vi "PFS_Telemetry.vi"(10 "Variant":variant) -> (2 "PFS_Telemetry":T1 {"Raw_Telemetry" format="%04x"; "Register_13"."Spare" format="%03x"})   [LabVIEW 2019, in "Variant Parser.lvlib" / "Variant Parser.lvclass"]
uses:
  Library/Variant Parser.lvclass
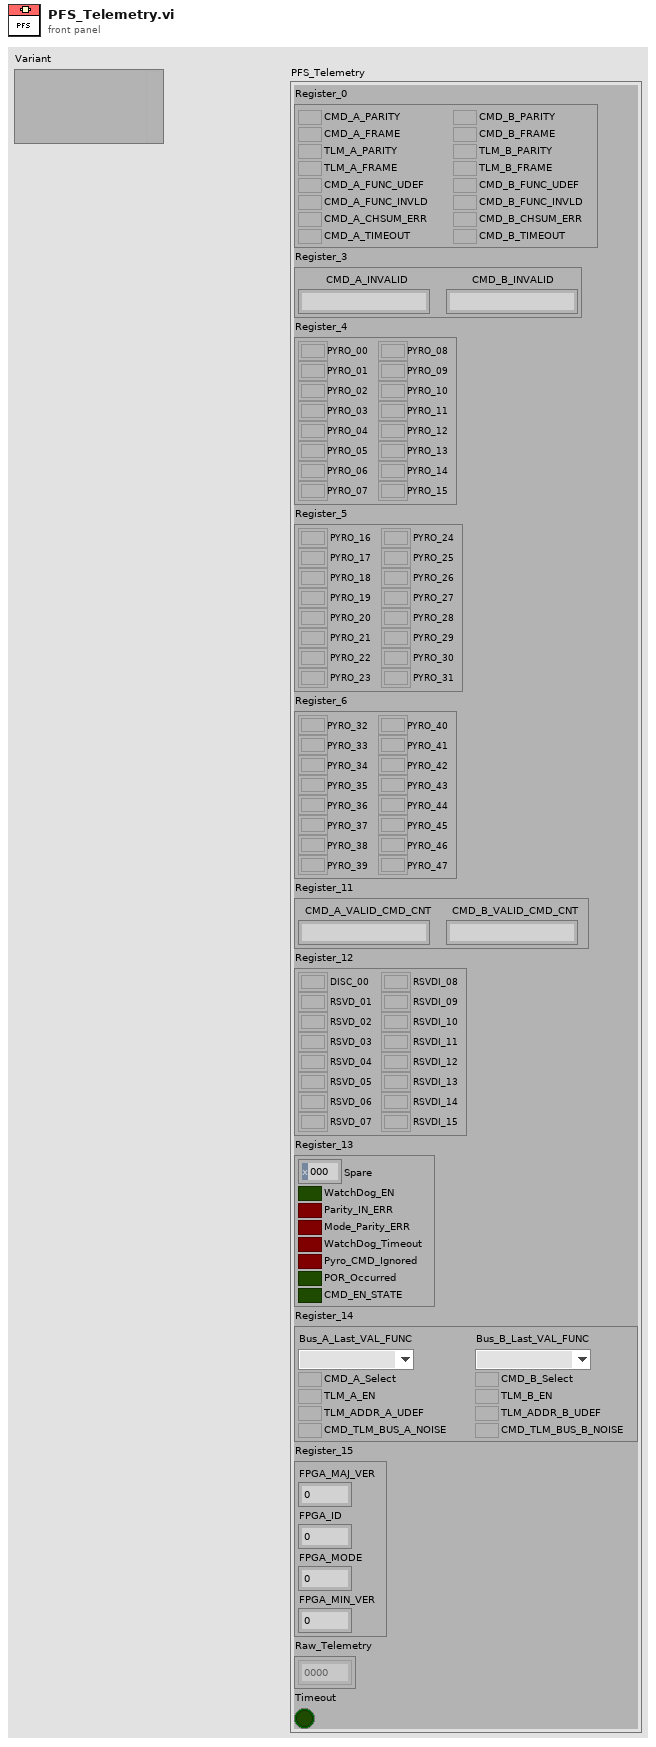
[diagram p1: front panel]
types:
  T1 = cluster{"Register_0":cluster{"CMD_B_PARITY":bool, "CMD_A_PARITY":bool, "CMD_B_FRAME":bool, "CMD_A_FRAME":bool, "TLM_B_PARITY":bool, "TLM_A_PARITY":bool, "TLM_B_FRAME":bool, "TLM_A_FRAME":bool, "CMD_B_FUNC_UDEF":bool, "CMD_A_FUNC_UDEF":bool, "CMD_B_FUNC_INVLD":bool, "CMD_A_FUNC_INVLD":bool, "CMD_B_CHSUM_ERR":bool, "CMD_A_CHSUM_ERR":bool, "CMD_B_TIMEOUT":bool, "CMD_A_TIMEOUT":bool}, "Register_3":cluster{"CMD_B_INVALID":u8, "CMD_A_INVALID":u8}, "Register_4":cluster{"PYRO_00":bool, "PYRO_01":bool, "PYRO_02":bool, "PYRO_03":bool, "PYRO_04":bool, "PYRO_05":bool, "PYRO_06":bool, "PYRO_07":bool, "PYRO_08":bool, "PYRO_09":bool, "PYRO_10":bool, "PYRO_11":bool, "PYRO_12":bool, "PYRO_13":bool, "PYRO_14":bool, "PYRO_15":bool}, "Register_5":cluster{"PYRO_16":bool, "PYRO_17":bool, "PYRO_18":bool, "PYRO_19":bool, "PYRO_20":bool, "PYRO_21":bool, "PYRO_22":bool, "PYRO_23":bool, "PYRO_24":bool, "PYRO_25":bool, "PYRO_26":bool, "PYRO_27":bool, "PYRO_28":bool, "PYRO_29":bool, "PYRO_30":bool, "PYRO_31":bool}, "Register_6":cluster{"PYRO_32":bool, "PYRO_33":bool, "PYRO_34":bool, "PYRO_35":bool, "PYRO_36":bool, "PYRO_37":bool, "PYRO_38":bool, "PYRO_39":bool, "PYRO_40":bool, "PYRO_41":bool, "PYRO_42":bool, "PYRO_43":bool, "PYRO_44":bool, "PYRO_45":bool, "PYRO_46":bool, "PYRO_47":bool}, "Register_11":cluster{"CMD_B_VALID_CMD_CNT":u8, "CMD_A_VALID_CMD_CNT":u8}, "Register_12":cluster{"DISC_00":bool, "RSVD_01":bool, "RSVD_02":bool, "RSVD_03":bool, "RSVD_04":bool, "RSVD_05":bool, "RSVD_06":bool, "RSVD_07":bool, "RSVDI_08":bool, "RSVDI_09":bool, "RSVDI_10":bool, "RSVDI_11":bool, "RSVDI_12":bool, "RSVDI_13":bool, "RSVDI_14":bool, "RSVDI_15":bool}, "Register_13":cluster{"Spare":u16, "WatchDog_EN":bool, "Parity_IN_ERR":bool, "Mode_Parity_ERR":bool, "WatchDog_Timeout":bool, "Pyro_CMD_Ignored":bool, "POR_Occurred":bool, "CMD_EN_STATE":bool}, "Register_14":cluster{"CMD_B_Select":bool, "CMD_A_Select":bool, "TLM_B_EN":bool, "TLM_A_EN":bool, "TLM_ADDR_B_UDEF":bool, "TLM_ADDR_A_UDEF":bool, "CMD_TLM_BUS_B_NOISE":bool, "CMD_TLM_BUS_A_NOISE":bool, "Bus_B_Last_VAL_FUNC":enum16{"No_Command", "IO_Command", "Pyro_Command", "Housekeeping", "Bad_Function"}, "Bus_A_Last_VAL_FUNC":enum16{"No_Command", "IO_Command", "Pyro_Command", "Housekeeping", "Bad_Function"}}, "Register_15":cluster{"FPGA_MAJ_VER":u8, "FPGA_ID":u8, "FPGA_MODE":u8, "FPGA_MIN_VER":u8}, "Raw_Telemetry":u16[], "Timeout":bool}
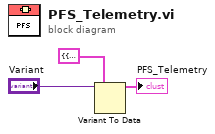
[diagram p0: block diagram]
diagram:
  n1 = Variant To Data(type=T1 {"Register_0"={"CMD_B_PARITY"=FALSE, "CMD_A_PARITY"=FALSE, "CMD_B_FRAME"=FALSE, "CMD_A_FRAME"=FALSE, "TLM_B_PARITY"=FALSE, "TLM_A_PARITY"=FALSE, "TLM_B_FRAME"=FALSE, "TLM_A_FRAME"=FALSE, "CMD_B_FUNC_UDEF"=FALSE, "CMD_A_FUNC_UDEF"=FALSE, "CMD_B_FUNC_INVLD"=FALSE, "CMD_A_FUNC_INVLD"=FALSE, "CMD_B_CHSUM_ERR"=FALSE, "CMD_A_CHSUM_ERR"=FALSE, "CMD_B_TIMEOUT"=FALSE, "CMD_A_TIMEOUT"=FALSE}, "Register_3"={"CMD_B_INVALID"=0, "CMD_A_INVALID"=0}, "Register_4"={"PYRO_00"=FALSE, "PYRO_01"=FALSE, "PYRO_02"=FALSE, "PYRO_03"=FALSE, "PYRO_04"=FALSE, "PYRO_05"=FALSE, "PYRO_06"=FALSE, "PYRO_07"=FALSE, "PYRO_08"=FALSE, "PYRO_09"=FALSE, "PYRO_10"=FALSE, "PYRO_11"=FALSE, "PYRO_12"=FALSE, "PYRO_13"=FALSE, "PYRO_14"=FALSE, "PYRO_15"=FALSE}, "Register_5"={"PYRO_16"=FALSE, "PYRO_17"=FALSE, "PYRO_18"=FALSE, "PYRO_19"=FALSE, "PYRO_20"=FALSE, "PYRO_21"=FALSE, "PYRO_22"=FALSE, "PYRO_23"=FALSE, "PYRO_24"=FALSE, "PYRO_25"=FALSE, "PYRO_26"=FALSE, "PYRO_27"=FALSE, "PYRO_28"=FALSE, "PYRO_29"=FALSE, "PYRO_30"=FALSE, "PYRO_31"=FALSE}, "Register_6"={"PYRO_32"=FALSE, "PYRO_33"=FALSE, "PYRO_34"=FALSE, "PYRO_35"=FALSE, "PYRO_36"=FALSE, "PYRO_37"=FALSE, "PYRO_38"=FALSE, "PYRO_39"=FALSE, "PYRO_40"=FALSE, "PYRO_41"=FALSE, "PYRO_42"=FALSE, "PYRO_43"=FALSE, "PYRO_44"=FALSE, "PYRO_45"=FALSE, "PYRO_46"=FALSE, "PYRO_47"=FALSE}, "Register_11"={"CMD_B_VALID_CMD_CNT"=0, "CMD_A_VALID_CMD_CNT"=0}, "Register_12"={"DISC_00"=FALSE, "RSVD_01"=FALSE, "RSVD_02"=FALSE, "RSVD_03"=FALSE, "RSVD_04"=FALSE, "RSVD_05"=FALSE, "RSVD_06"=FALSE, "RSVD_07"=FALSE, "RSVDI_08"=FALSE, "RSVDI_09"=FALSE, "RSVDI_10"=FALSE, "RSVDI_11"=FALSE, "RSVDI_12"=FALSE, "RSVDI_13"=FALSE, "RSVDI_14"=FALSE, "RSVDI_15"=FALSE}, "Register_13"={"Spare"=0, "WatchDog_EN"=FALSE, "Parity_IN_ERR"=FALSE, "Mode_Parity_ERR"=FALSE, "WatchDog_Timeout"=FALSE, "Pyro_CMD_Ignored"=FALSE, "POR_Occurred"=FALSE, "CMD_EN_STATE"=FALSE}, "Register_14"={"CMD_B_Select"=FALSE, "CMD_A_Select"=FALSE, "TLM_B_EN"=FALSE, "TLM_A_EN"=FALSE, "TLM_ADDR_B_UDEF"=FALSE, "TLM_ADDR_A_UDEF"=FALSE, "CMD_TLM_BUS_B_NOISE"=FALSE, "CMD_TLM_BUS_A_NOISE"=FALSE, "Bus_B_Last_VAL_FUNC"=enum."No_Command", "Bus_A_Last_VAL_FUNC"=enum."No_Command"}, "Register_15"={"FPGA_MAJ_VER"=0, "FPGA_ID"=0, "FPGA_MODE"=0, "FPGA_MIN_VER"=0}, "Raw_Telemetry"=[], "Timeout"=FALSE} ("PFS_Telemetry"), Variant="Variant") -> (data=→"PFS_Telemetry":T1)  [unwired: 1 in, 1 out]
